vi "Actual PID.vi"(8 "Current Input":dbl, 11 "Wanted End":dbl) -> (3 "Output":dbl)   [LabVIEW 2017]
panel:
  in  "PID Speed":dbl=0.43
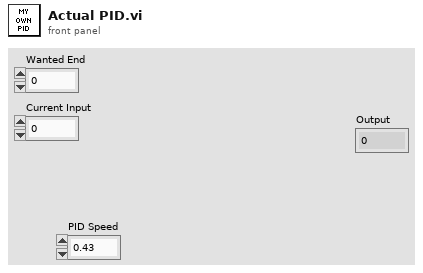
[diagram p1: front panel]
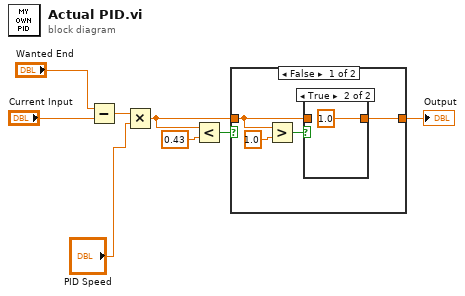
[diagram p0: block diagram]
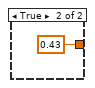
[diagram p3: hidden frame]
diagram:
  n1 = Subtract(x="Wanted End", y="Current Input") -> (x-y=w6:dbl)
  n2 = Multiply(x=w6, y="PID Speed") -> (x*y=w2:dbl)
  n3 = Less?(x=w2, y=0.43) -> (x < y?=w5:bool)
  n4 = case shown="False" w5 {
    tunnel: [w9 0.43 ("y")] -> w3
    tunnel: w2 -> [w10 _]
    frame False {
      n5 = Greater?(x=w10, y=1.0) -> (0:w12:bool)
      n6 = case shown="True" w12 {
        tunnel: w10 -> [w13 _]
        tunnel: [w13 1.0 ("y")] -> w9
        frame False {
        }
        frame True {
        }
      }
    }
    frame True {
    }
  }
  "Output" <- w3
